vi "Action Update Ramp Rate-with-queue-teardown.vi"(8 "error out":errorcluster) -> (3 "result":bool)   [LabVIEW 2018]
uses:
  Libraries/Thermal Chamber Response Simulator/Thermal Chamber Response Simulator.lvlib
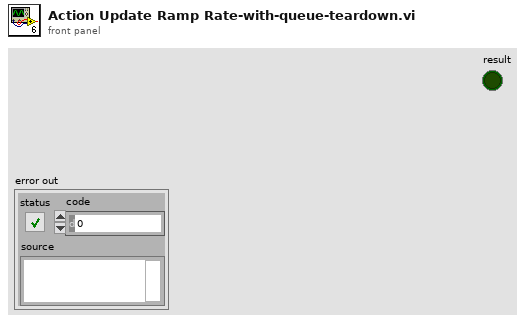
[diagram p1: front panel]
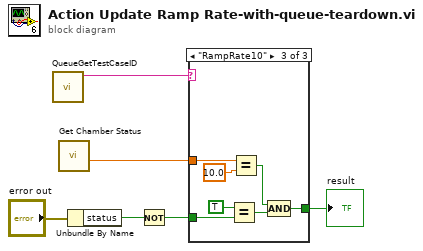
[diagram p0: block diagram]
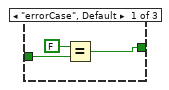
[diagram p2: hidden frame]
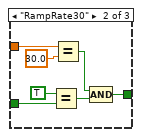
[diagram p3: hidden frame]
diagram:
  n1 = call "QueueGetTestCaseID.vi"() -> ("test case ID"=w1:string)  [unwired: 11 in]
  n2 = call "Get Chamber Status.vi"() -> ("Ramp Rate (deg C / second)"=w2:dbl)  [unwired: 6 in, 5 out]
  n3 = Unbundle By Name("error out") -> ("status"=w6:bool)
  n4 = Not(x=w6) -> (.not. x?=w4:bool)
  n5 = case shown="\"RampRate10\"" w1 {
    tunnel: w4 -> [w7 w11 w23]
    tunnel: w2 -> [_ w12 w20]
    tunnel: [w8 w10 w17] -> w3
    frame "errorCase", Default {
      n6 = Equal?(x=FALSE, y=w7) -> (x = y?=w8:bool)
    }
    frame "RampRate30" {
      n7 = Equal?(x=TRUE, y=w11) -> (x = y?=w13:bool)
      n8 = Equal?(x=w12, y=30.0) -> (x = y?=w14:bool)
      n9 = Compound Arithmetic op=AND(w14, w13) -> (w10:bool)
    }
    frame "RampRate10" {
      n10 = Equal?(x=TRUE, y=w23) -> (x = y?=w18:bool)
      n11 = Equal?(x=w20, y=10.0) -> (x = y?=w19:bool)
      n12 = Compound Arithmetic op=AND(w19, w18) -> (w17:bool)
    }
  }
  "result" <- w3
